vi "obtain image queue.vi"(8 "error in (no error)":errorcluster, 11 "DAQCascade512II in":refnum<class "DAQCascade512II.lvclass">) -> (0 "error out":errorcluster, 3 "DAQCascade512II out":refnum<class "DAQCascade512II.lvclass">)   [LabVIEW 2012, in "DAQCascade512II.lvclass"]
uses:
  DAQCascade512II.lvclass
  DAQCascade512II.lvclass/DAQCascade512II.ctl
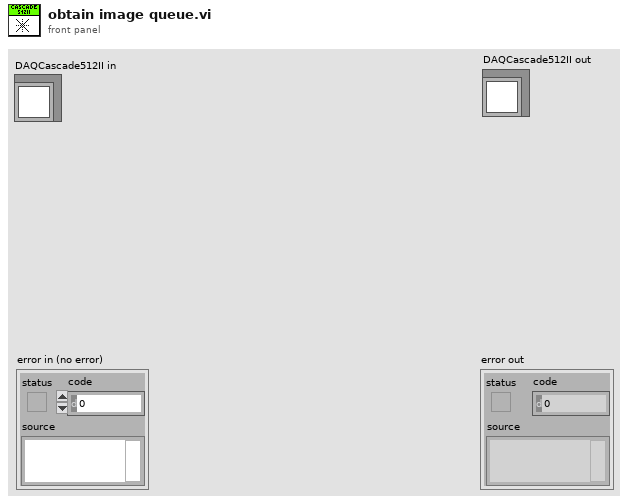
[diagram p1: front panel]
types:
  T1 = cluster{"Array uint 16":u16[][], "setting.File Path":path}
  T2 = typedef "Image Type" = u32
  T3 = typedef "IMAQ Image.ctl" = refnum<image>
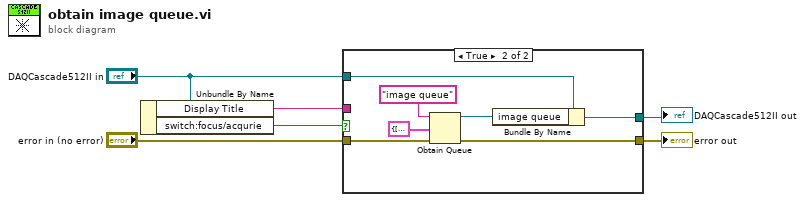
[diagram p0: block diagram]
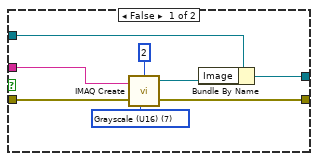
[diagram p2: hidden frame]
diagram:
  n1 = Unbundle By Name("DAQCascade512II in") -> ("Display Title"=w1:string, "switch:focus/acqurie"=w2:bool)
  n2 = case shown="True" w2 {
    tunnel: "error in (no error)" -> [w12 w19]
    tunnel: [w11 w18] -> w5
    tunnel: "DAQCascade512II in" -> [w9 w17]
    tunnel: [w8 w15] -> w4
    tunnel: w1 -> [w7 _]
    frame False {
      w14 = T2 7 items=["Grayscale (U8)", "Grayscale (I16)", "Grayscale (SGL)", "Complex (CSG)", "RGB (U32)", "HSL (U32)", "RGB (U64)", "Grayscale (U16)"] ("Image Type")
      n3 = call "IMAQ Create"("Border Size"=2, "Image Name"=w7, "Image Type"=w14, "error in (no error)"=w12) -> ("New Image"=w10:T3, "error out"=w11:errorcluster)  [unwired: 1 in]
      n4 = Bundle By Name(cluster=w9, "Image"=w10) -> (w8:refnum<class "DAQCascade512II.lvclass">)
    }
    frame True {
      n5 = Obtain Queue(name (unnamed)="image queue", element data type=T1 {"Array uint 16"=[], "setting.File Path"=path ""}, error in (no error)=w19) -> (queue out=w16:refnum<queue>, error out=w18:errorcluster)  [unwired: 2 in, 1 out]
      n6 = Bundle By Name(cluster=w17, "image queue"=w16) -> (w15:refnum<class "DAQCascade512II.lvclass">)
    }
  }
  "error out" <- w5
  "DAQCascade512II out" <- w4
